vi "IsMaster.vi"(8 "error in (no error)":errorcluster, 11 "Network Protocol in":refnum<class "Network Protocol.lvclass">) -> (0 "error out":errorcluster, 2 "isMaster":bool, 3 "Network Protocol out":refnum<class "Network Protocol.lvclass">)   [LabVIEW 2021, in "Network Protocol.lvclass"]
uses:
  Network Protocol.lvclass
  Network Protocol.lvclass/Network Protocol.ctl
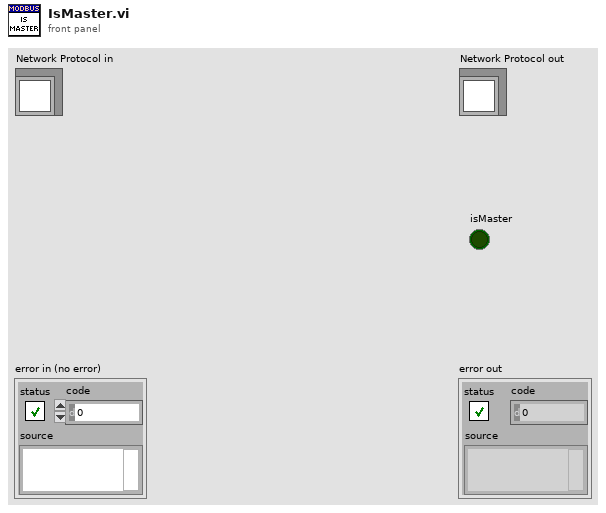
[diagram p1: front panel]
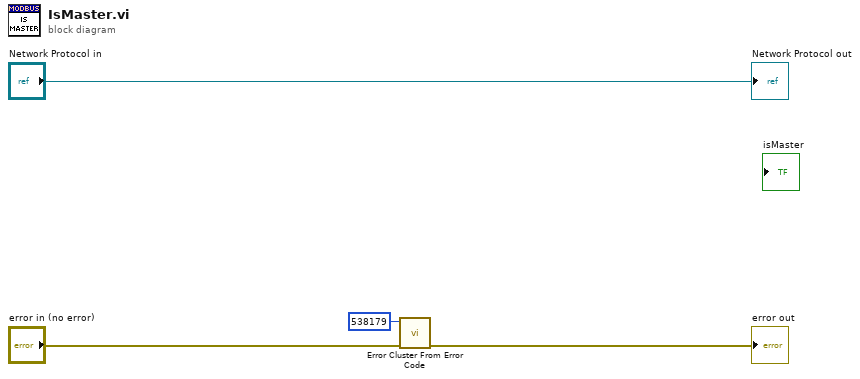
[diagram p0: block diagram]
diagram:
  n1 = call <vilib>:"Error Cluster From Error Code.vi"("error in (no error)"="error in (no error)", "error code (0)"=538179) -> ("error out"=→"error out":errorcluster)  [unwired: 7 in]
  "Network Protocol out" <- "Network Protocol in"
